vi "get last byte.vi"(11 "EthernetIP Channel in":refnum<class "EthernetIP Channel.lvclass">) -> (3 "last byte":i32)   [LabVIEW 2013, in "EthernetIP Channel.lvclass"]
uses:
  EthernetIP Channel.lvclass
  <vilib>/NI/Tag Bus/tag/tag descriptor.lvclass/tag descriptor.ctl
  EthernetIP Channel.lvclass/EthernetIP Channel.ctl
  <vilib>/NI/Tag Bus/tag/tag descriptor.lvclass
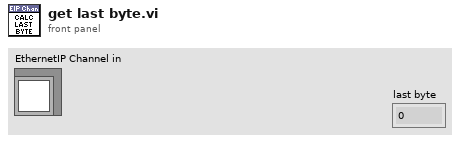
[diagram p1: front panel]
types:
  T1 = typedef "tag bus.lvlib/tag descriptor.lvclass/Data Type.ctl" = enum16{"Double", "Single", "I64", "I32", "I16", "I8", "U64", "U32", "U16", "U8", "Boolean", "String", "Array of Double", "Array of Single", "Array of I64", "Array of I32", "Array of I16", "Array of I8", "Array of U64", "Array of U32", "Array of U16", "Array of U8", "Array of Boolean", "Array of String"}
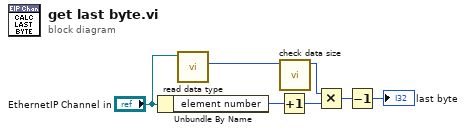
[diagram p0: block diagram]
diagram:
  n1 = Unbundle By Name("EthernetIP Channel in") -> ("element number"=w4:i32)
  n2 = call <vilib>:"read data type.vi"("system tag in"="EthernetIP Channel in") -> ("data type"=w6:T1)  [unwired: 8 in, 2 out]
  n3 = Increment(x=w4) -> (x+1=w1:i32)
  n4 = call "check data size.vi"("data type"=w6) -> ("bytes"=w5:i32)  [unwired: 10 in]
  n5 = Multiply(x=w5, y=w1) -> (x*y=w3:i32)
  n6 = Decrement(x=w3) -> (x-1=→"last byte":i32)
